vi "dfd_DFXP Sub (ss).vi"(5 "quantize output?(T)":bool=TRUE, 7 "op params":T6={"source"=0, "is floating?"=FALSE, "o-mode"=enum."Wrap", "q-mode"=enum."Truncation", "wl"=1, "high limit"=0, "low limit"=0, "iwl"=0, "sign?"=TRUE} {"source" items=["Coef a/k"=0, "Coef b/v"=7, "Input"=1, "Output"=2, "Multiplicand"=3, "Product"=4, "Sum"=5, "Delay"=6, "Gain"=8]}, 8 "filtering statistics in":T5(array[cluster]) {"statistics information"."min value" format="%.2f"; "statistics information"."max value" format="%.2f"; "Quantizer Source" items=["Coefficients a/k"=0, "Coefficients b/v"=7, "Input"=1, "Output"=2, "Multiplicand"=3, "Product"=4, "Sum"=5, "Delay"=6]}, 10 "Value in 2":T1={"value"=0, "wl"=0, "iwl"=0, "Signed"=TRUE} {"value" format="%.0x"}, 11 "Value in":T1={"value"=0, "wl"=0, "iwl"=0, "Signed"=TRUE} {"value" format="%.0x"}) -> (0 "filtering statistics out":T5(array[cluster]) {"statistics information"."min value" format="%.2f"; "statistics information"."max value" format="%.2f"; "Quantizer Source" items=["Coefficients a/k"=0, "Coefficients b/v"=7, "Input"=1, "Output"=2, "Multiplicand"=3, "Product"=4, "Sum"=5, "Delay"=6]}, 3 "Value out":T1={"value"=0, "wl"=0, "iwl"=0, "Signed"=TRUE} {"value" format="%.0x"})   [LabVIEW 2017, in "NI_DigFilter_FXP.lvlib"]
uses:
  <vilib>/addons/Digital Filter Design/NI_DigFilter_FXP.lvlib
  <vilib>/addons/Digital Filter Design/_Objects.llb/dfd_DFXP Data Type (scaler).ctl
  <vilib>/addons/Digital Filter Design/_Objects.llb/dfd_DFXP Operation Parameter.ctl
  <vilib>/addons/Digital Filter Design/_Objects.llb/dfd_Internal Quantization Srcs.ctl
  <vilib>/addons/Digital Filter Design/_Objects.llb/DFD Quantization Sources.ctl
  <vilib>/addons/Digital Filter Design/_Objects.llb/DFD FXP Statistics Data.ctl
  <vilib>/addons/Digital Filter Design/_Objects.llb/dfd_DFXP Data Type 128bits (scaler).ctl
  <vilib>/addons/Digital Filter Design/NI_DigFilterLicensed.lvlib
panel:
  in  "Value type":T1={"value"=0, "wl"=0, "iwl"=0, "Signed"=TRUE} {"value" format="%.0x"}
  in  "Value type":T2 {"Low 64" format="%.0x"; "High 64" format="%.0x"}
  in  "Value type64":T1={"value"=0, "wl"=0, "iwl"=0, "Signed"=TRUE} {"value" format="%.0x"}
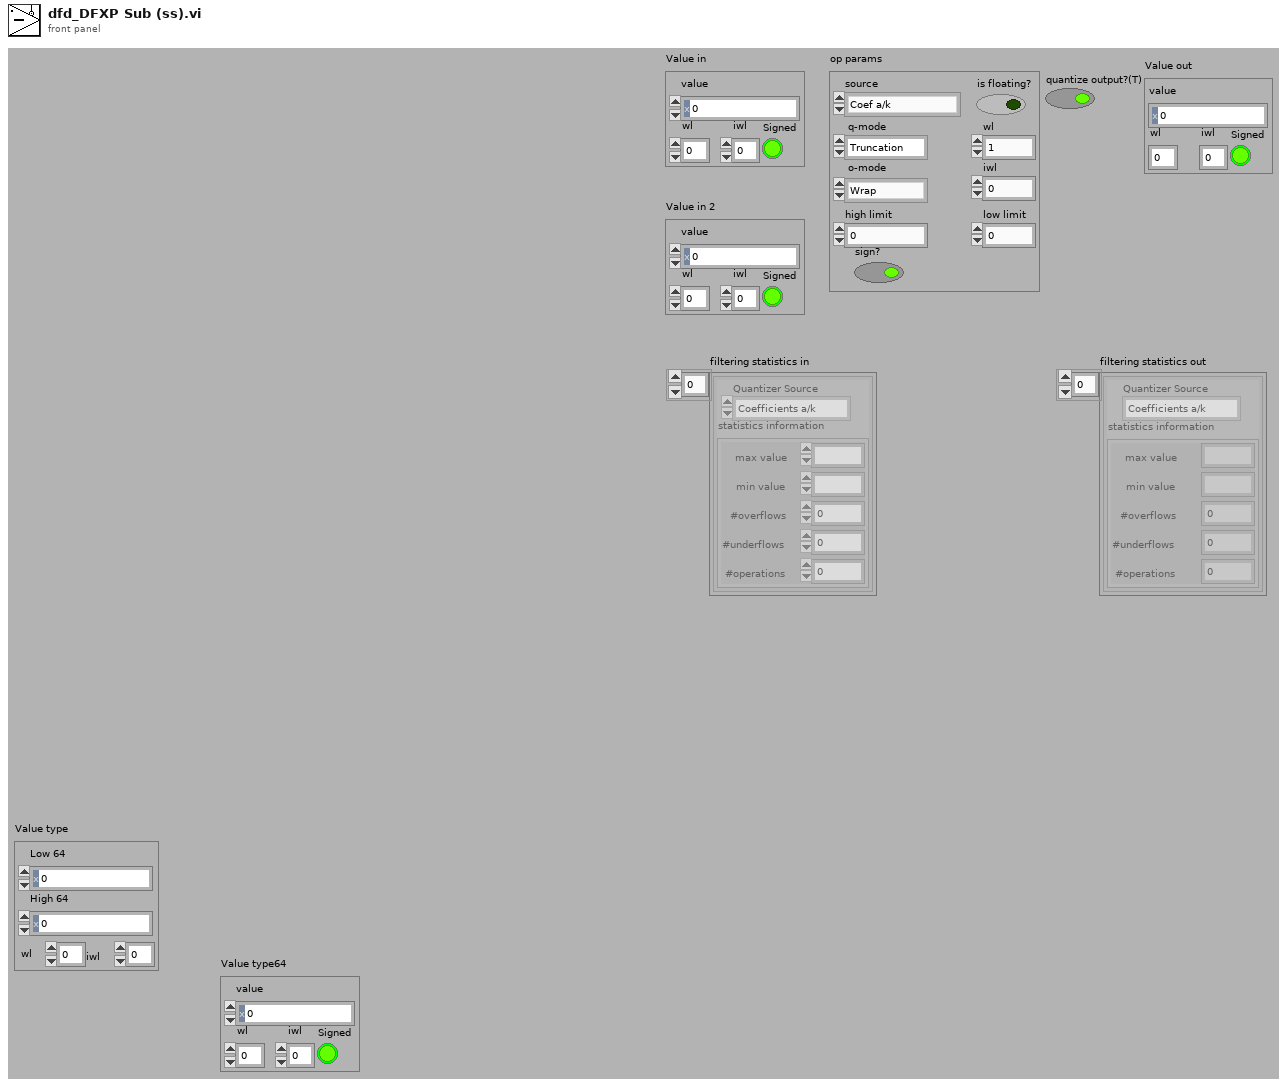
[diagram p1: front panel]
types:
  T1 = typedef "dfd_DFXP Data Type (scaler).ctl" = cluster{"value":i64, "wl":i16, "iwl":i16, "Signed":bool}
  T2 = typedef "dfd_DFXP Data Type 128bits (scaler).ctl" = cluster{"Low 64":u64, "High 64":i64, "wl":i16, "iwl":i16}
  T3 = typedef "NI_DigFilterLicensed.lvlib/DFD Quantization Sources.ctl" = u16
  T4 = typedef "NI_DigFilterLicensed.lvlib/DFD FXP Statistics Data.ctl" = cluster{"max value":ext, "min value":ext, "#overflows":i32, "#underflows":i32, "#operations":i32}
  T5 = cluster{"Quantizer Source":T3, "statistics information":T4}[]
  T6 = typedef "dfd_DFXP Operation Parameter.ctl" = cluster{"source":T7, "is floating?":bool, "o-mode":enum16{"Saturation", "Wrap"}, "q-mode":enum16{"Nearest", "Truncation"}, "wl":i16, "high limit":i64, "low limit":i64, "iwl":i16, "sign?":bool}
  T7 = typedef "NI_DigFilterLicensed.lvlib/dfd_Internal Quantization Srcs.ctl" = u16
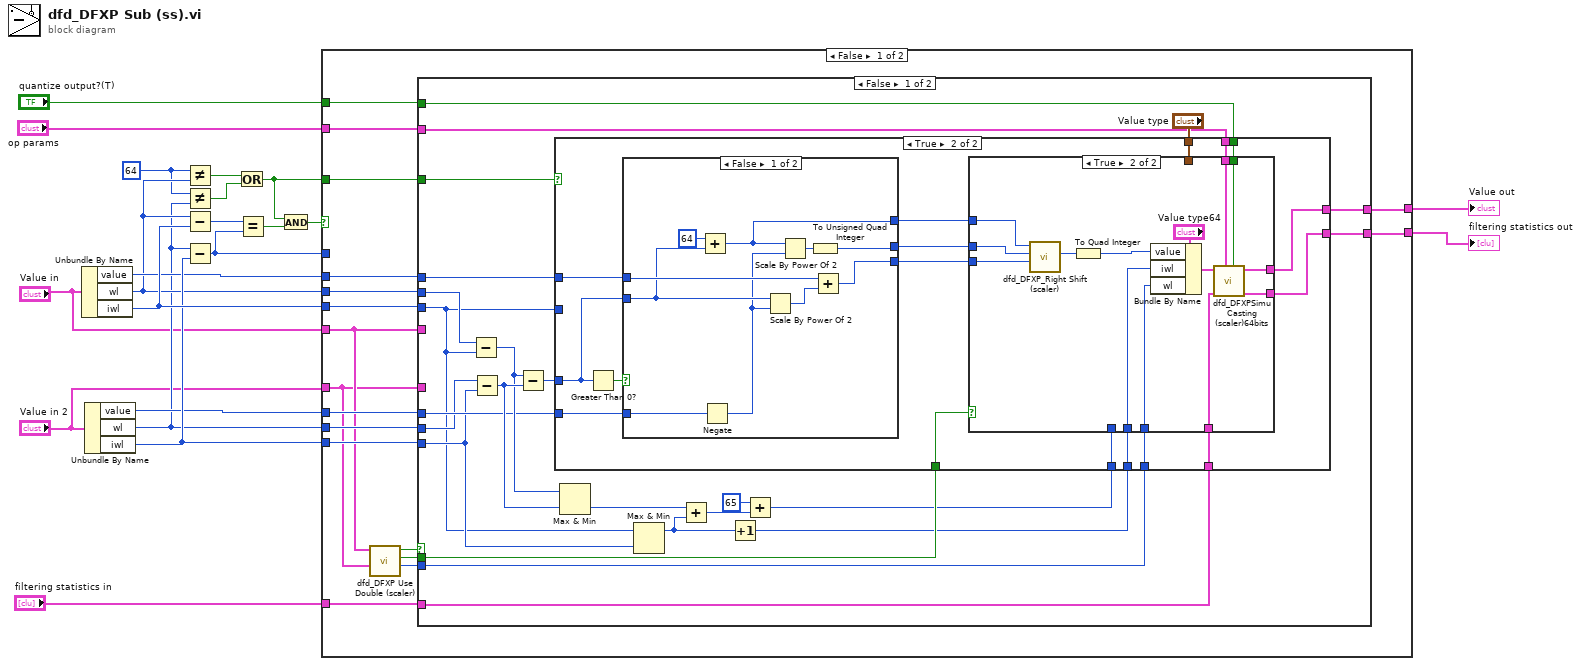
[diagram p0: block diagram]
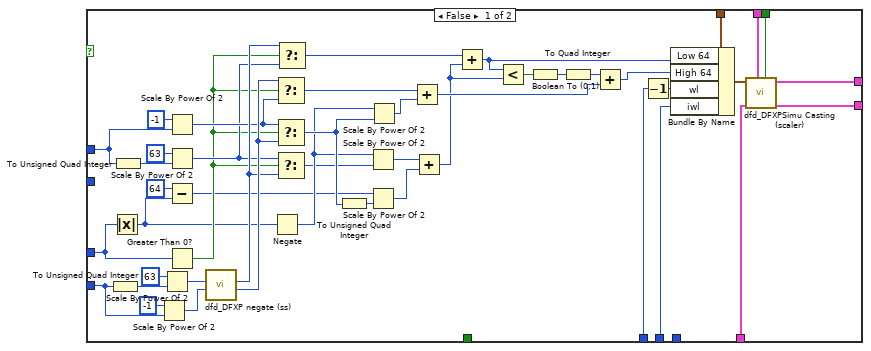
[diagram p2: hidden frame]
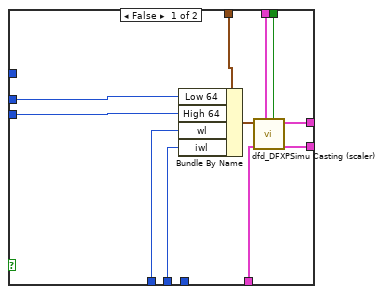
[diagram p3: hidden frame]
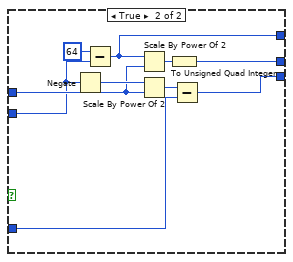
[diagram p4: hidden frame]
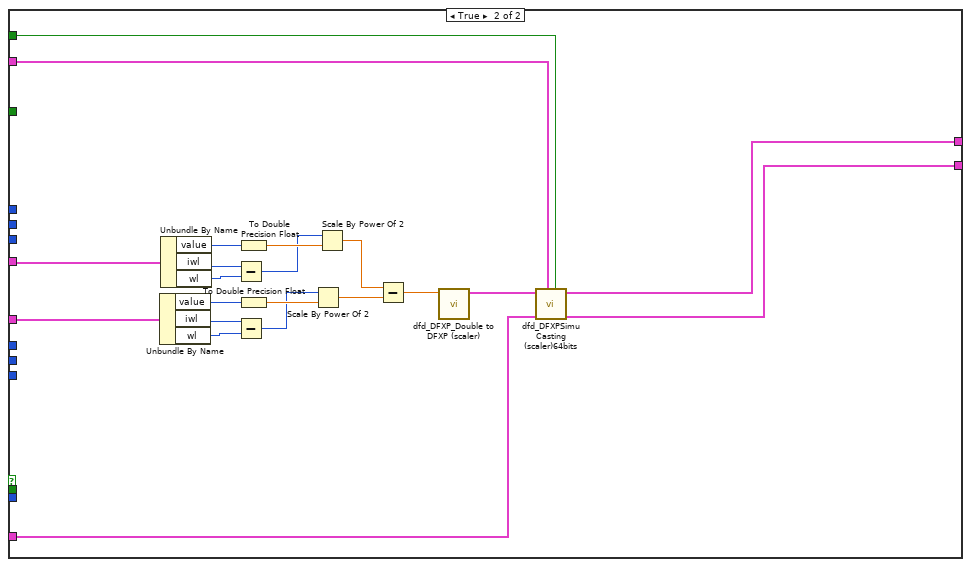
[diagram p5: hidden frame]
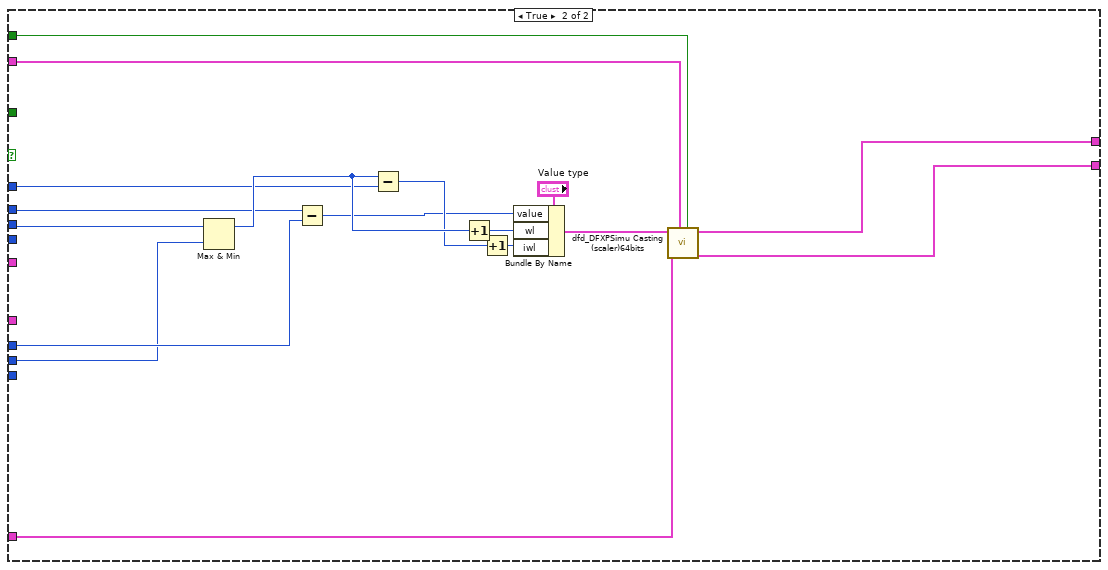
[diagram p6: hidden frame]
diagram:
  w10 = i16 64 ("y")
  n1 = Unbundle By Name("Value in") -> ("value"=w19:i64, "wl"=w12:i16, "iwl"=w21:i16)
  n2 = Unbundle By Name("Value in 2") -> ("value"=w18:i64, "wl"=w11:i16, "iwl"=w20:i16)
  n3 = Not Equal?(x=w10, y=w12) -> (x != y?=w13:bool)
  n4 = Not Equal?(x=w10, y=w11) -> (x != y?=w9:bool)
  n5 = Subtract(x=w12, y=w21) -> (x-y=w17:i16)
  n6 = Subtract(x=w11, y=w20) -> (x-y=w16:i16)
  n7 = Or(x=w13, y=w9) -> (x .or. y?=w8:bool)
  n8 = Equal?(x=w17, y=w16) -> (x = y?=w15:bool)
  n9 = And(x=w8, y=w15) -> (x .and. y?=w14:bool)
  n10 = case shown="False" w14 {
    tunnel: w12 -> [w35 w196]
    tunnel: w21 -> [w34 _]
    tunnel: w11 -> [w32 w194]
    tunnel: w20 -> [w31 _]
    tunnel: w18 -> [w33 w195]
    tunnel: w19 -> [w36 w197]
    tunnel: "Value in" -> [w26 _]
    tunnel: "Value in 2" -> [w25 _]
    tunnel: "filtering statistics in" -> [w30 w193]
    tunnel: "op params" -> [w37 w199]
    tunnel: [w28 w191] -> w1
    tunnel: [w29 w192] -> w2
    tunnel: "quantize output?(T)" -> [w38 w200]
    tunnel: w16 -> [_ w198]
    tunnel: w8 -> [w27 _]
    frame False {
      n11 = call <vilib>:"dfd_DFXP Use Double (scaler).vi"("Value in 2"=w25, "Value in"=w26) -> ("Result wl"=w22:i16, "Use 64?"=w23:bool, "Use double?"=w24:bool)  [unwired: 7 out]
      n12 = case shown="False" w24 {
        tunnel: [w45 w186] -> w28
        tunnel: w30 -> [w46 w188]
        tunnel: [w44 w187] -> w29
        tunnel: w37 -> [w43 w185]
        tunnel: w36 -> [w56 _]
        tunnel: w35 -> [w55 _]
        tunnel: w34 -> [w39 _]
        tunnel: w33 -> [w54 _]
        tunnel: w32 -> [w53 _]
        tunnel: w31 -> [w52 _]
        tunnel: w38 -> [w42 w184]
        tunnel: w26 -> [_ w180]
        tunnel: w25 -> [_ w175]
        tunnel: w27 -> [w51 _]
        tunnel: w23 -> [w50 _]
        tunnel: w22 -> [w40 _]
        frame False {
          n13 = Subtract(x=w55, y=w39) -> (x-y=w58:i16)
          n14 = Subtract(x=w53, y=w52) -> (x-y=w62:i16)
          n15 = Subtract(x=w58, y=w62) -> (x-y=w41:i16)
          n16 = Max & Min(x=w58, y=w62) -> (min(x,y)=w61:i16)  [unwired: 1 out]
          n17 = Max & Min(x=w39, y=w52) -> (max(x,y)=w57:i16)  [unwired: 1 out]
          n18 = Add(x=w61, y=w57) -> (x+y=w60:i16)
          n19 = Increment(x=w57) -> (x+1=w47:i16)
          n20 = Add(x=i16 65, y=w60) -> (x+y=w48:i16)
          n21 = case shown="True" w51 {
            tunnel: w41 -> [w66 w121]
            tunnel: w56 -> [w67 w123]
            tunnel: w54 -> [w65 w122]
            tunnel: w50 -> [_ w118]
            tunnel: "Value type" -> [w104 w117]
            tunnel: w48 -> [w106 w116]
            tunnel: w47 -> [w105 w115]
            tunnel: w46 -> [w103 w114]
            tunnel: [w99 w113] -> w45
            tunnel: [w100 w112] -> w44
            tunnel: w43 -> [w102 w111]
            tunnel: w42 -> [w101 w110]
            tunnel: w40 -> [_ w108]
            tunnel: w39 -> [_ _]
            frame False {
              n22 = To Unsigned Quad Integer(1:w65) -> (0:w73:u64)
              n23 = Absolute Value(x=w66) -> (abs(x)=w76:i16)
              n24 = To Unsigned Quad Integer(1:w67) -> (0:w72:u64)
              n25 = Scale By Power Of 2(n=-1, x=w65) -> (x*2^n=w95:i64)
              n26 = Scale By Power Of 2(n=63, x=w73) -> (x*2^n=w94:u64)
              n27 = Scale By Power Of 2(n=-1, x=w67) -> (x*2^n=w93:i64)
              n28 = Scale By Power Of 2(n=63, x=w72) -> (x*2^n=w83:u64)
              n29 = Subtract(x=i16 64, y=w76) -> (x-y=w69:i16)
              n30 = Greater Than 0?(x=w66) -> (x > 0?=w82:bool)
              n31 = call <vilib>:"dfd_DFXP negate (ss).vi"("High 64"=w95, "Low 64"=w94) -> ("High 64"=w97:i64, "Low 64"=w96:u64)  [unwired: 8 out]
              n32 = Negate(x=w76) -> (-x=w79:i16)
              n33 = Select(t=w97, s=w82, f=w93) -> (s? t:f=w85:i64)
              n34 = Select(t=w93, s=w82, f=w97) -> (s? t:f=w81:i64)
              n35 = Select(t=w83, s=w82, f=w96) -> (s? t:f=w78:u64)
              n36 = Select(t=w96, s=w82, f=w83) -> (s? t:f=w86:u64)
              n37 = To Unsigned Quad Integer(1:w81) -> (0:w77:u64)
              n38 = Scale By Power Of 2(n=w79, x=w78) -> (x*2^n=w92:u64)
              n39 = Scale By Power Of 2(n=w69, x=w77) -> (x*2^n=w80:u64)
              n40 = Scale By Power Of 2(n=w79, x=w81) -> (x*2^n=w84:i64)
              n41 = Add(x=w85, y=w84) -> (x+y=w90:i64)
              n42 = Add(x=w92, y=w80) -> (x+y=w87:u64)
              n43 = Add(x=w86, y=w87) -> (x+y=w64:u64)
              n44 = Less?(x=w64, y=w87) -> (x < y?=w88:bool)
              n45 = Boolean To (0,1)(Boolean=w88) -> (0, 1=w89:i16)
              n46 = To Quad Integer(1:w89) -> (0:w91:i64)
              n47 = Add(x=w91, y=w90) -> (x+y=w63:i64)
              n48 = Decrement(x=w106) -> (x-1=w98:i16)
              n49 = Bundle By Name(cluster=w104, "Low 64"=w64, "High 64"=w63, "wl"=w98, "iwl"=w105) -> (w107:T2)
              n50 = call <vilib>:"dfd_DFXPSimu Casting (scaler).vi"("quantize output? (T)"=w101, "op params"=w102, "filtering statistics in"=w103, "Value in"=w107) -> ("filtering statistics out"=w99:T5, "Value out"=w100:T1)  [unwired: 6 out]
            }
            frame True {
              n51 = Greater Than 0?(x=w121) -> (x > 0?=w124:bool)
              n52 = case shown="False" w124 {
                tunnel: [w152 w161] -> w120
                tunnel: [w151 w163] -> w119
                tunnel: w123 -> [w155 w166]
                tunnel: w122 -> [w156 w160]
                tunnel: w121 -> [w154 w165]
                tunnel: [w153 w162] -> w109
                frame False {
                  n53 = Add(x=i16 64 ("y"), y=w154) -> (x+y=w153:i16)
                  n54 = Negate(x=w156) -> (-x=w150:i64)
                  n55 = Scale By Power Of 2(n=w154, x=w150) -> (x*2^n=w157:i64)
                  n56 = Scale By Power Of 2(n=w153, x=w150) -> (x*2^n=w158:i64)
                  n57 = To Unsigned Quad Integer(1:w158) -> (0:w152:u64)
                  n58 = Add(x=w155, y=w157) -> (x+y=w151:i64)
                }
                frame True {
                  n59 = Negate(x=w165) -> (-x=w168:i16)
                  n60 = Subtract(x=i16 64 ("y"), y=w165) -> (x-y=w162:i16)
                  n61 = Scale By Power Of 2(n=w162, x=w166) -> (x*2^n=w167:i64)
                  n62 = Scale By Power Of 2(n=w168, x=w166) -> (x*2^n=w164:i64)
                  n63 = To Unsigned Quad Integer(1:w167) -> (0:w161:u64)
                  n64 = Subtract(x=w164, y=w160) -> (x-y=w163:i64)
                }
              }
              n65 = case shown="True" w118 {
                tunnel: w120 -> [w133 w148]
                tunnel: w119 -> [w132 w147]
                tunnel: w117 -> [w134 _]
                tunnel: w116 -> [w131 _]
                tunnel: w115 -> [w130 w142]
                tunnel: w114 -> [w129 w140]
                tunnel: [w128 w138] -> w113
                tunnel: [w127 w137] -> w112
                tunnel: w111 -> [w126 w146]
                tunnel: w110 -> [w125 w136]
                tunnel: w109 -> [_ w149]
                tunnel: w108 -> [_ w141]
                frame False {
                  n66 = Bundle By Name(cluster=w134, "Low 64"=w133, "High 64"=w132, "wl"=w131, "iwl"=w130) -> (w135:T2)
                  n67 = call <vilib>:"dfd_DFXPSimu Casting (scaler).vi"("quantize output? (T)"=w125, "op params"=w126, "filtering statistics in"=w129, "Value in"=w135) -> ("filtering statistics out"=w128:T5, "Value out"=w127:T1)  [unwired: 6 out]
                }
                frame True {
                  n68 = call <vilib>:"dfd_DFXP_Right Shift (scaler).vi"("High 64"=w147, "Low 64"=w148, "Num"=w149) -> ("Low 64"=w144:u64)  [unwired: 8 out]
                  n69 = To Quad Integer(1:w144) -> (0:w143:i64)
                  n70 = Bundle By Name(cluster="Value type64", "value"=w143, "iwl"=w142, "wl"=w141) -> (w139:T1)
                  n71 = call <vilib>:"dfd_DFXPSimu Casting (scaler)64bits.vi"("quantize output?(T)"=w136, "op params"=w146, "filtering statistics in"=w140, "Value in"=w139) -> ("filtering statistics out"=w138:T5, "Value out"=w137:T1)  [unwired: 6 out]
                }
              }
            }
          }
        }
        frame True {
          n72 = Unbundle By Name(w175) -> ("value"=w177:i64, "iwl"=w173:i16, "wl"=w174:i16)
          n73 = Unbundle By Name(w180) -> ("value"=w182:i64, "iwl"=w171:i16, "wl"=w170:i16)
          n74 = Subtract(x=w171, y=w170) -> (x-y=w181:i16)
          n75 = Subtract(x=w173, y=w174) -> (x-y=w176:i16)
          n76 = To Double Precision Float(number=w182) -> (double precision float=w183:dbl)
          n77 = To Double Precision Float(number=w177) -> (double precision float=w178:dbl)
          n78 = Scale By Power Of 2(n=w176, x=w178) -> (x*2^n=w172:dbl)
          n79 = Scale By Power Of 2(n=w181, x=w183) -> (x*2^n=w179:dbl)
          n80 = Subtract(x=w179, y=w172) -> (x-y=w190:dbl)
          n81 = call <vilib>:"dfd_DFXP_Double to DFXP (scaler).vi"("Double"=w190) -> ("FXP"=w189:T1)  [unwired: 10 out]
          n82 = call <vilib>:"dfd_DFXPSimu Casting (scaler)64bits.vi"("quantize output?(T)"=w184, "op params"=w185, "filtering statistics in"=w188, "Value in"=w189) -> ("filtering statistics out"=w186:T5, "Value out"=w187:T1)  [unwired: 6 out]
        }
      }
    }
    frame True {
      n83 = Max & Min(x=w196, y=w194) -> (max(x,y)=w206:i16)  [unwired: 1 out]
      n84 = Subtract(x=w197, y=w195) -> (x-y=w202:i64)
      n85 = Subtract(x=w206, y=w198) -> (x-y=w205:i16)
      n86 = Increment(x=w206) -> (x+1=w203:i16)
      n87 = Increment(x=w205) -> (x+1=w204:i16)
      n88 = Bundle By Name(cluster="Value type", "value"=w202, "wl"=w203, "iwl"=w204) -> (w201:T1)
      n89 = call <vilib>:"dfd_DFXPSimu Casting (scaler)64bits.vi"("quantize output?(T)"=w200, "op params"=w199, "filtering statistics in"=w193, "Value in"=w201) -> ("filtering statistics out"=w191:T5, "Value out"=w192:T1)  [unwired: 6 out]
    }
  }
  "Value out" <- w2
  "filtering statistics out" <- w1
